vi "Apply UserPwd DB Config Obj.vi"(8 "error in (no error)":errorcluster, 10 "UserPwd DB Configuration Obj":refnum<class "UserPwd DB Configuration.lvclass">, 11 "VacuumLines Configuration in":refnum<class "VacuumLines Configuration.lvclass">) -> (0 "error out":errorcluster, 3 "VacuumLines Configuration out":refnum<class "VacuumLines Configuration.lvclass">)   [LabVIEW 2016, in "Hardware.lvlib" / "VacuumLine.lvlib" / "VacuumLines Configuration.lvclass"]
uses:
  <userlib>/Common Components/Hardware/Abstract System/VacuumLine/VacuumLines Configuration/VacuumLines Configuration.lvclass
  <userlib>/Common Components/UserPwd DB/UserPwd DB Config/UserPwd DB Configuration.lvclass
  <userlib>/Common Components/Hardware/Abstract System/VacuumLine/VacuumLines Configuration/VacuumLines Configuration.lvclass/VacuumLines Configuration.ctl
  <userlib>/Common Components/UserPwd DB/UserPwd DB Config/UserPwd DB Configuration.lvclass/UserPwd DB Configuration.ctl
  <userlib>/Common Components/Hardware/Abstract System/VacuumLine/VacuumLines/VacuumLines.lvclass
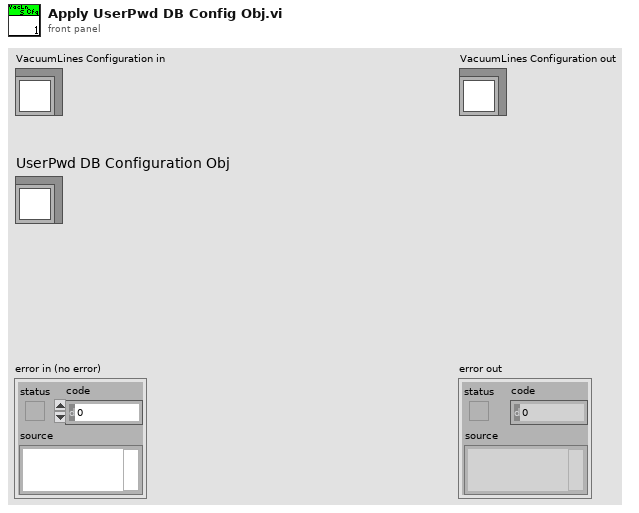
[diagram p1: front panel]
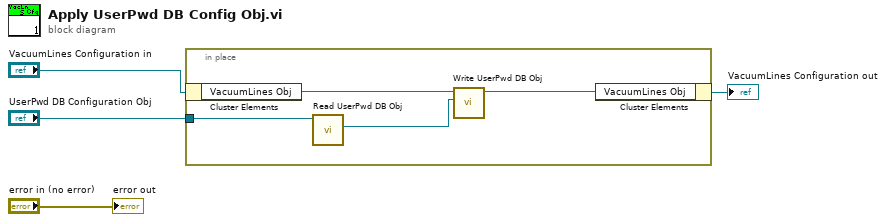
[diagram p0: block diagram]
diagram:
  n1 = in-place {
    in-place-border: "UserPwd DB Configuration Obj" -> [w8]
    n2 = in-place-cluster #1("VacuumLines Configuration in") -> ("VacuumLines Obj"=w7:refnum<class "VacuumLines.lvclass">)
    n3 = call <userlib>:"Read UserPwd DB Obj.vi"("UserPwd DB Configuration in"=w8) -> ("UserPwd DB.lvlib:UserPwd DB.lvclass"=w5:refnum<class "UserPwd DB.lvclass">)  [unwired: 9 in, 1 out]
    n4 = call <userlib>:"Write UserPwd DB Obj.vi"("UserPwd DB.lvlib:UserPwd DB.lvclass"=w5, "VacuumLines in"=w7) -> ("VacuumLines out"=w6:refnum<class "VacuumLines.lvclass">)  [unwired: 9 in]
    n5 = in-place-cluster #1("VacuumLines Obj"=w6) -> (→"VacuumLines Configuration out":refnum<class "VacuumLines Configuration.lvclass">)
  }
  "error out" <- "error in (no error)"
